vi "Remove Sink.vi"(6 "Remove all matches? (F)":bool, 8 "Error In":errorcluster, 10 "Name":string, 11 "Logger in":refnum<class "Log.lvclass">) -> (0 "Error Out":errorcluster, 3 "Logger":refnum<class "Log.lvclass">)   [LabVIEW 2019, in "TSC Event Logger.lvlib" / "Log.lvclass"]
doc: "Remove the named sink from the list.\n\n<b>Code Developed By:</b>\nTechnology Service Corporation\nBloomington, IN 47403\nwww.tsc.com/atcs\n\nDeveloper:\nDaniel Coons"
uses:
  Log.lvclass
  Log.lvclass/Log.ctl
  Log Sinks/Log Sinks.lvclass/Log Sinks.ctl
  Log Sinks/Log Sinks.lvclass
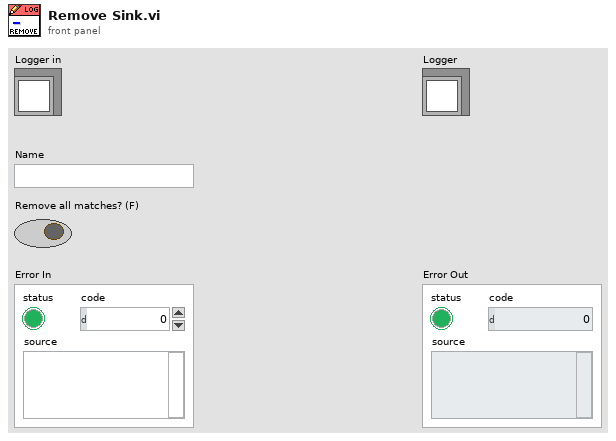
[diagram p1: front panel]
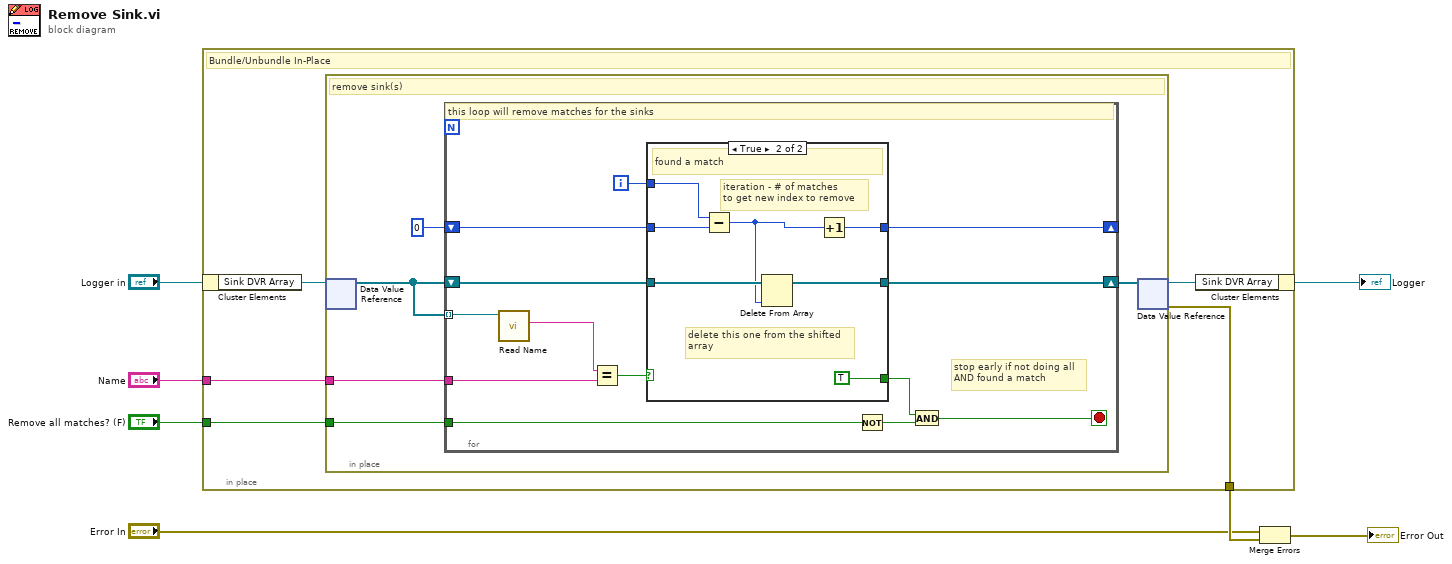
[diagram p0: block diagram]
diagram:
  n1 = in-place {
    in-place-border: [w10] -> w4
    in-place-border: "Name" -> [w9]
    in-place-border: "Remove all matches? (F)" -> [w8]
    # "Bundle/Unbundle In-Place"
    n2 = in-place-cluster #1("Logger in") -> ("Sink DVR Array"=w12:refnum<data-value>)
    n3 = in-place {
      in-place-border: w9 -> [w17]
      in-place-border: w8 -> [w16]
      # "remove sink(s)"
      n4 = in-place-dvr #2(w12) -> (w15:refnum<class "Log Sinks.lvclass">[])  [unwired: 1 out]
      n5 = for {
        tunnel: w15 -> [w30] mode=indexing
        tunnel: w17 -> [w28]
        tunnel: w16 -> [w18]
        shift-right: [w26] -> w14
        shift-left: w15 -> [w27]
        shift-right: [w23] -> _
        shift-left: 0 -> [w24]
        i -> [w25]
        stop <- w20 stop-if-true
        # "stop early if not doing all\nAND found a match"
        # "this loop will remove matches for the sinks"
        n6 = call "Read Name.vi"("Log Sinks in"=w30) -> ("Name"=w29:string)  [unwired: 9 in, 1 out]
        n7 = Equal?(x=w29, y=w28) -> (x = y?=w22:bool)
        n8 = case shown="True" w22 {
          tunnel: w27 -> [w31 w39]
          tunnel: [w31 w38] -> w26
          tunnel: w25 -> [_ w37]
          tunnel: w24 -> [w32 w36]
          tunnel: [w32 w34] -> w23
          tunnel: [_ TRUE] -> w19
          frame False {
            # "not a match"
          }
          frame True {
            # "delete this one from the shifted\narray"
            # "iteration - # of matches \nto get new index to remove"
            # "found a match"
            n9 = Subtract(x=w37, y=w36) -> (x-y=w35:i32)
            n10 = Delete From Array "Delete From Array"(array=w39, index=w35) -> (array with subset deleted=w38:refnum<class "Log Sinks.lvclass">[])  [unwired: 1 in, 1 out]
            n11 = Increment(x=w35) -> (x+1=w34:i32)
          }
        }
        n12 = Not(x=w18) -> (.not. x?=w21:bool)
        n13 = And(x=w19, y=w21) -> (x .and. y?=w20:bool)
      }
      n14 = in-place-dvr #2(w14) -> (w11:refnum<data-value>, w10:errorcluster)
    }
    n15 = in-place-cluster #1("Sink DVR Array"=w11) -> (→"Logger":refnum<class "Log.lvclass">)
  }
  n16 = Merge Errors("Error In", w4) -> (→"Error Out":errorcluster)
